vi "ClosestPoint.vi"(6 "Reset":bool, 8 "Robot":cluster{"x":dbl, "y":dbl}, 11 "Path":cluster{"x":dbl, "y":dbl}[](array[cluster])) -> (2 "ClosestIndex":i32, 3 "Point":cluster{"x":dbl, "y":dbl})   [LabVIEW 2017]
doc: "Find the closest point to the robot"
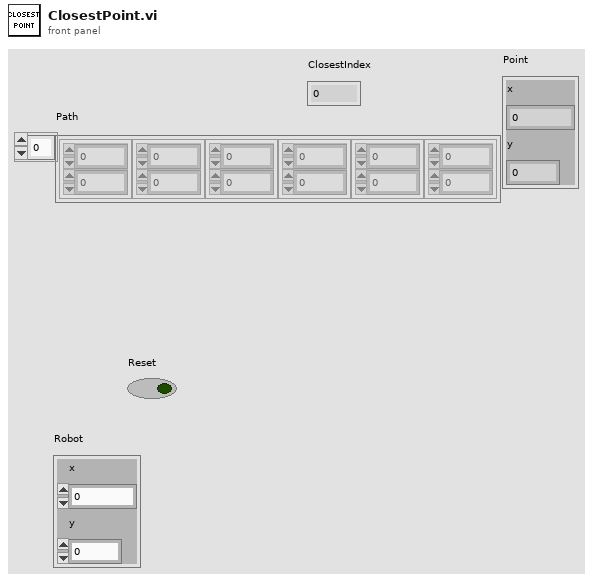
[diagram p1: front panel]
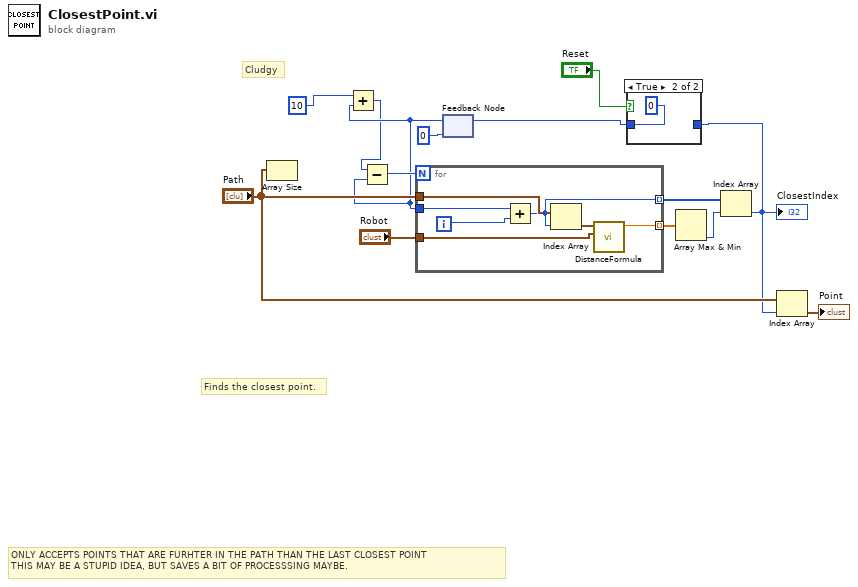
[diagram p0: block diagram]
diagram:
  # "Cludgy"
  # "ONLY ACCEPTS POINTS THAT ARE FURHTER IN THE PATH THAN THE LAST CLOSEST POINT\nTHIS MAY BE A STUPID IDEA, BUT SAVES A BIT OF PROCESSSING MAYBE."
  # "Finds the closest point."
  n1 = Array Size(array="Path") -> ()  [unwired: 1 out]
  n2 = feedback #1(0) -> (w5:i32)
  n3 = Add(x=10, y=w5) -> (x+y=w4:i32)
  n4 = Subtract(x=w4, y=w5) -> (x-y=w10:i32)
  n5 = for {
    N: w10 -> [_]
    tunnel: "Path" -> [w20]
    tunnel: "Robot" -> [w21]
    tunnel: w5 -> [w19]
    tunnel: [w17] -> w8 mode=indexing
    tunnel: [w16] -> w9 mode=indexing
    i -> [w15]
    n6 = Add(x=w19, y=w15) -> (x+y=w17:i32)
    n7 = Index Array(array=w20, index=w17) -> (element=w18:cluster{"x":dbl, "y":dbl})
    n8 = call "DistanceFormula.vi"("Point 2"=w21, "Point 1"=w18) -> ("Distance"=w16:dbl)  [unwired: 9 in]
  }
  n9 = Array Max & Min(array=w9) -> (min index (indices)=w7:i32)  [unwired: 3 out]
  n10 = Index Array(array=w8, index=w7) -> (element=w2:i32)
  "ClosestIndex" <- w2
  n11 = case shown="True" "Reset" {
    tunnel: w2 -> [w22 _]
    tunnel: [w22 0] -> w1
    frame False {
    }
    frame True {
    }
  }
  n12 = feedback-in #1(w1) -> ()
  n13 = Index Array(array="Path", index=w2) -> (element=→"Point":cluster{"x":dbl, "y":dbl})
